vi "CreateImage.vi"() -> ()   [LabVIEW 2020]
panel:
  in  "NumTriangles":i32
  in  "NumImages":i32
  in  "CreateNegImages":bool
  in  "CreatePosImages":bool
  in  "ExportNeg":bool
  in  "NumOvals":i32
  in  "NumRectangles":i32
  in  "stop":bool
  in  "ExportPos":bool
  in  "CreateImage":bool
  out "height":dbl
  out "y":dbl
  out "width":dbl
  out "x":dbl
  out "2D Picture":picture
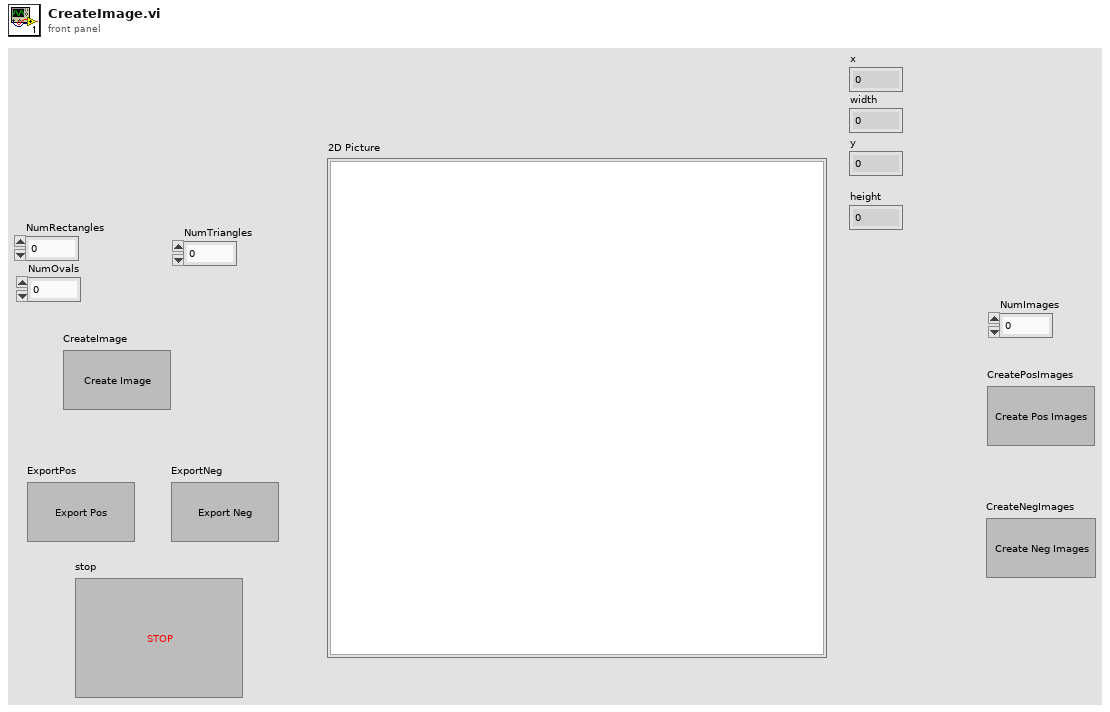
[diagram p1: front panel]
types:
  T1 = cluster{"left":i16, "top":i16, "right":i16, "bottom":i16}
  T2 = enum16{"open", "replace", "create", "open or create", "replace or create", "replace or create with confirmation"}
  T3 = cluster{"Width":u16, "Style":enum32{"Solid", "Dash", "Dot", "DashDot", "DashDotDot"}}
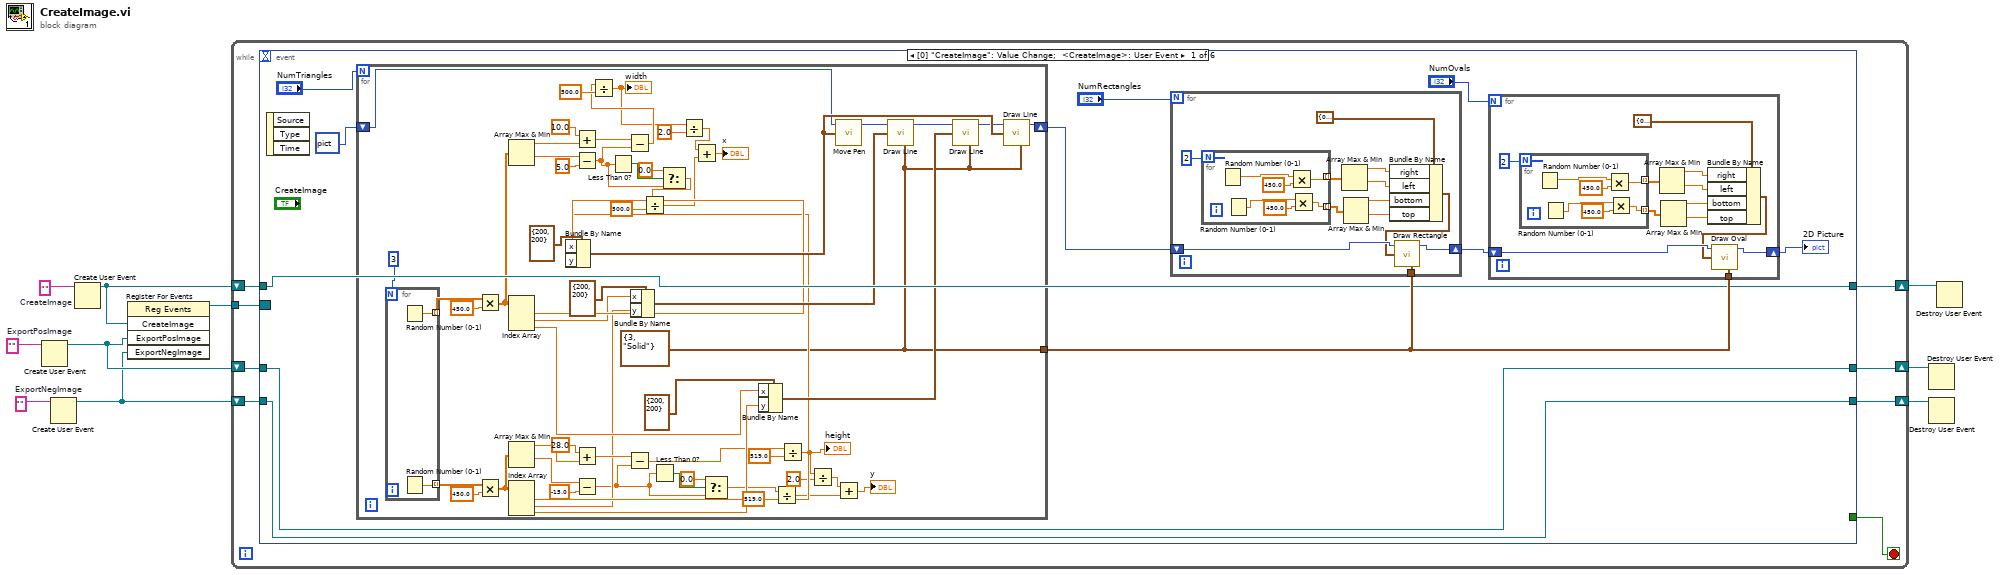
[diagram p0: block diagram]
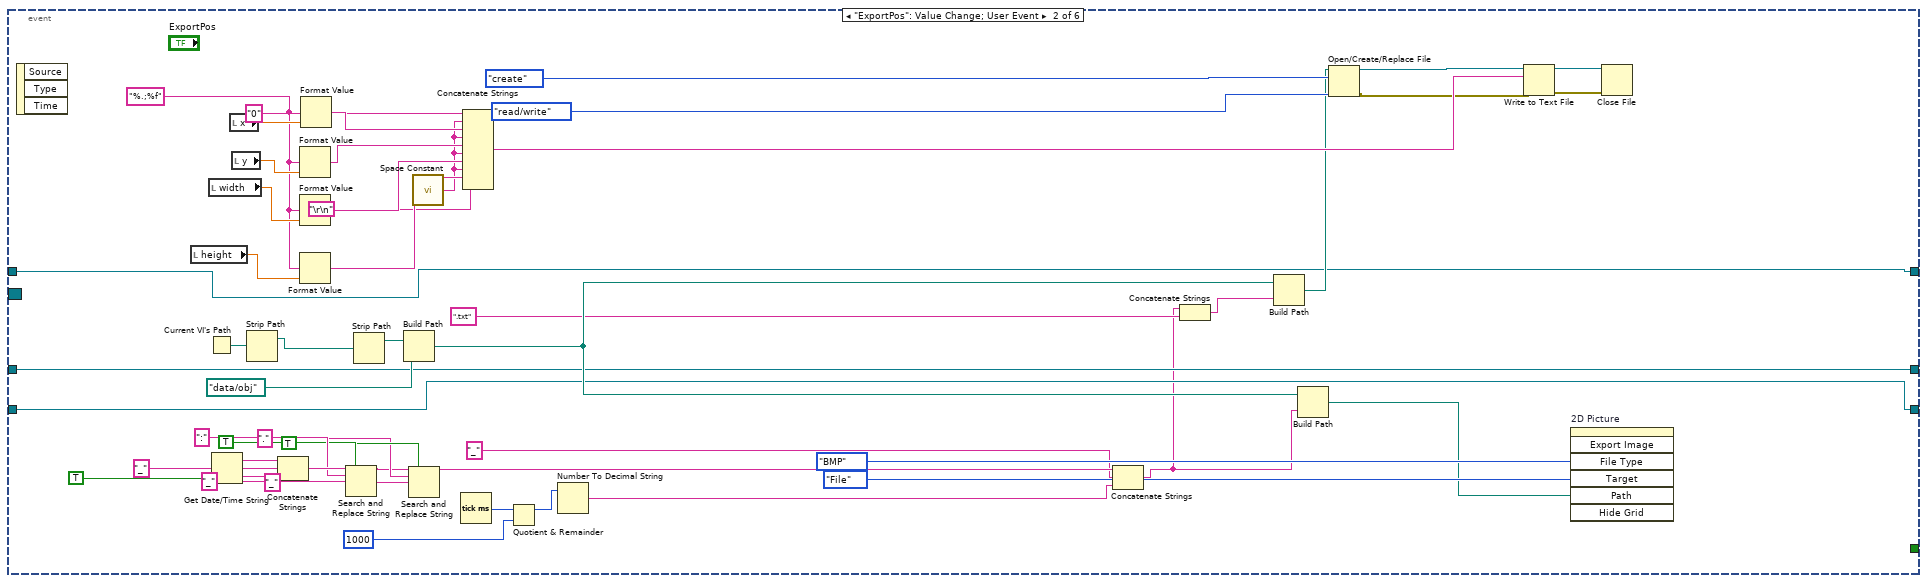
[diagram p2: hidden frame]
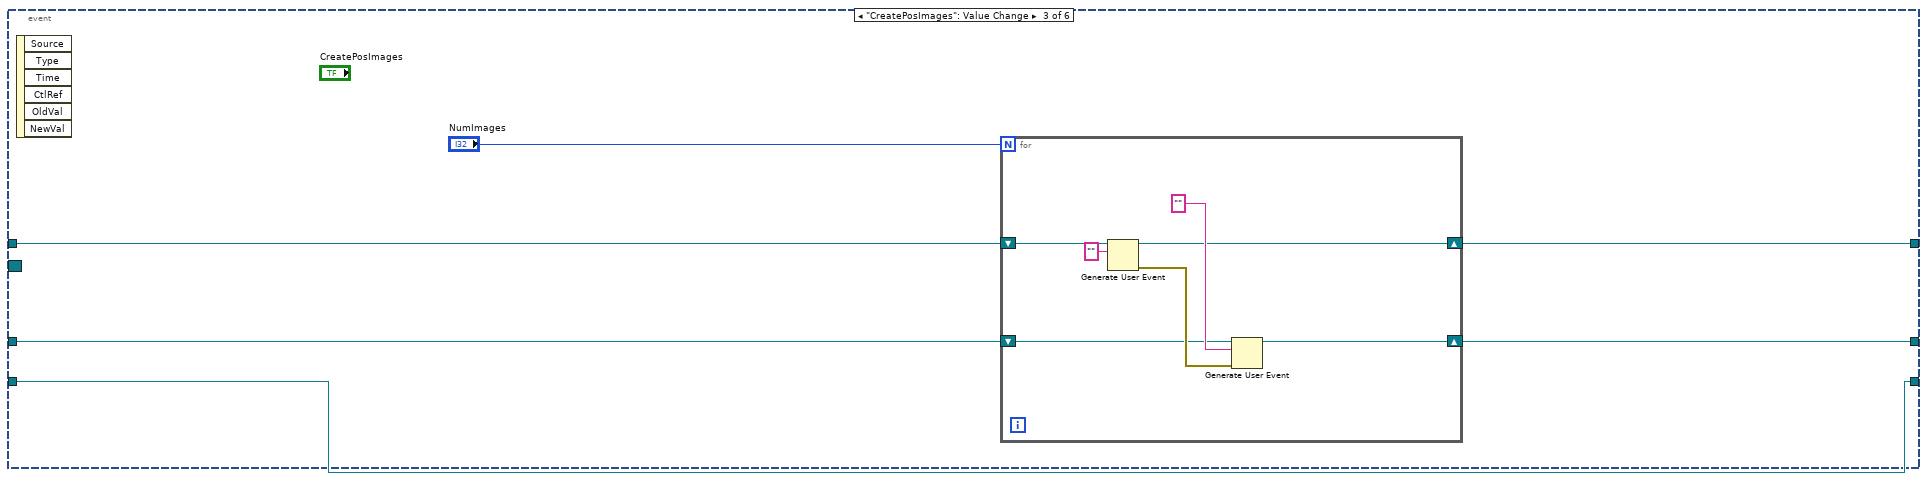
[diagram p3: hidden frame]
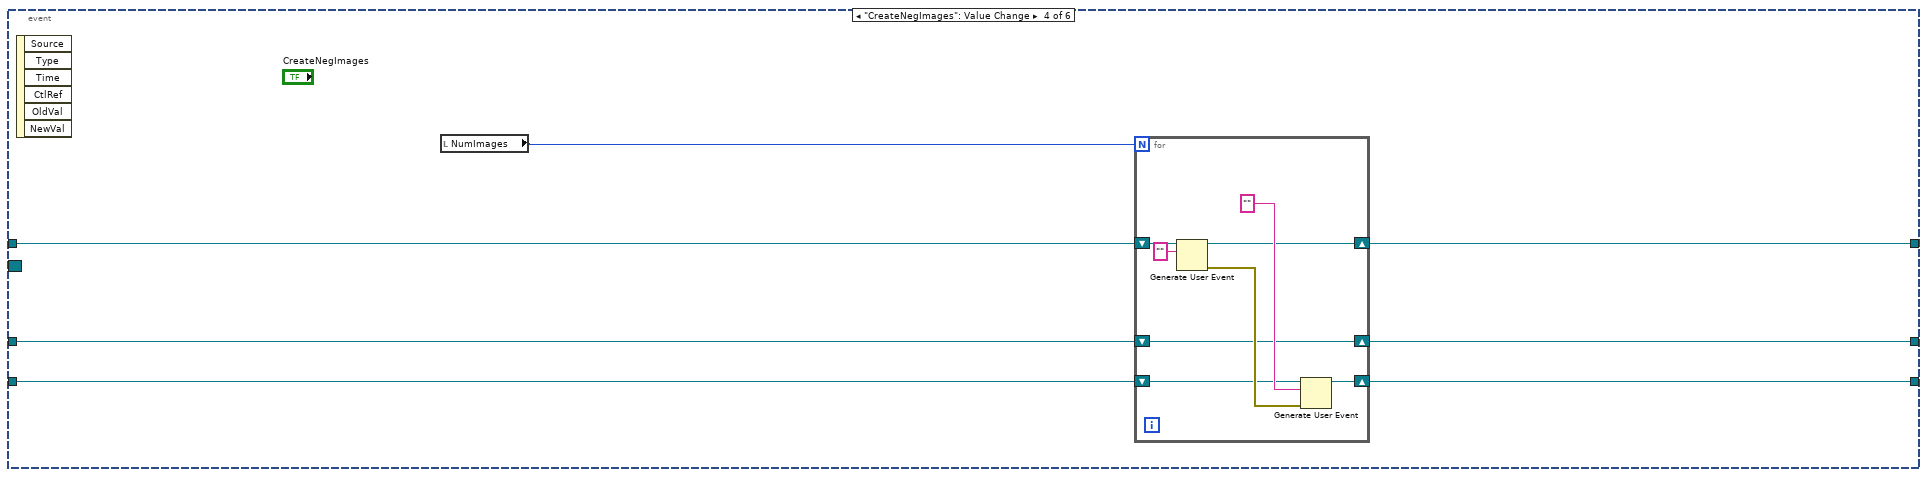
[diagram p4: hidden frame]
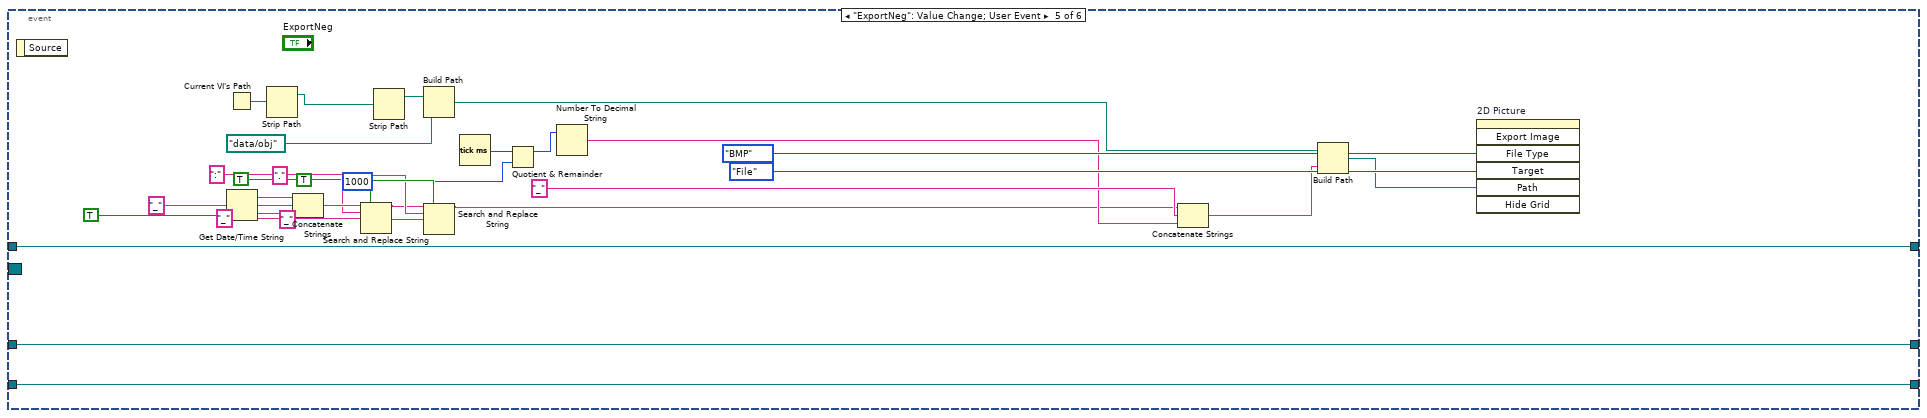
[diagram p5: hidden frame]
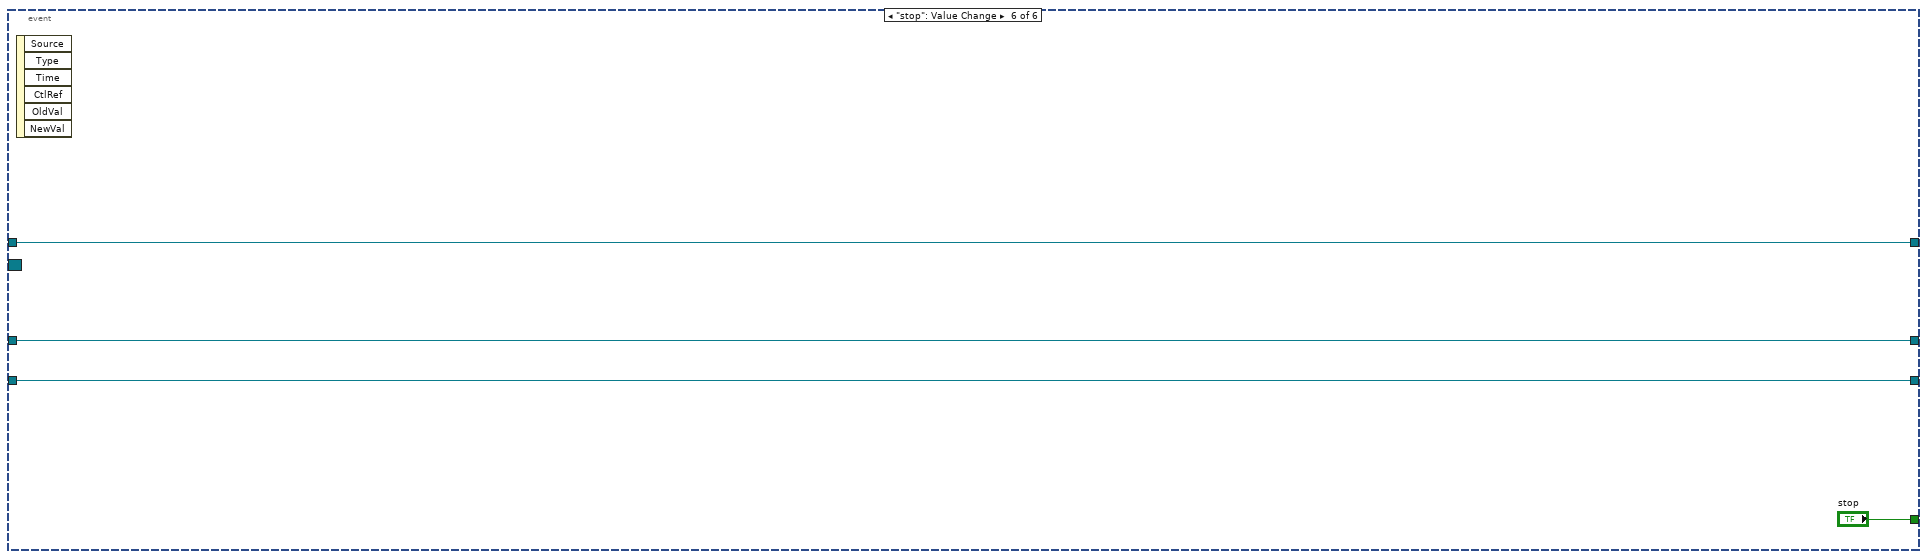
[diagram p6: hidden frame]
diagram:
  w4 = ""  # ExportNegImage
  w6 = ""  # ExportPosImage
  w10 = ""  # CreateImage
  n1 = Create User Event(user event datatype=w6) -> (user event=w5:refnum<user-event>)  [unwired: 1 in, 1 out]
  n2 = Create User Event(user event datatype=w4) -> (user event=w3:refnum<user-event>)  [unwired: 1 in, 1 out]
  n3 = Create User Event(user event datatype=w10) -> (user event=w8:refnum<user-event>)  [unwired: 1 in, 1 out]
  n4 = register-events(w8, w5, w3) -> (reference out=w9:refnum<event-registration>)  [unwired: 2 in, 1 out]
  n5 = while {
    tunnel: w9 -> [w17]
    shift-right: [w15] -> w7
    shift-left: w8 -> [w16]
    shift-right: [w13] -> w2
    shift-left: w5 -> [w14]
    shift-right: [w11] -> w1
    shift-left: w3 -> [w12]
    stop <- w18 stop-if-true
    n6 = event shown="[0] \"CreateImage\": Value Change;  <CreateImage>: User Event" {
      selector: w17 -> [_ _ _ _ _ _]
      dyn-events: _ -> [_ _ _ _ _ _]
      timeout: _ -> [_ _ _ _ _ _]
      tunnel: [_ _ _ _ _ "stop"] -> w18
      tunnel: w16 -> [w23 w134 w184 w198 w216 w239]
      tunnel: [w23 w134 w183 w197 w216 w239] -> w15
      tunnel: w14 -> [w24 w135 w181 w195 w215 w238]
      tunnel: [w24 w135 w182 w196 w215 w238] -> w13
      tunnel: w12 -> [w25 w136 w180 w194 w214 w237]
      tunnel: [w25 w136 w180 w193 w214 w237] -> w11
      event "CreateImage": Value Change; User Event {
        n7 = event-data() -> ()  [unwired: 1 in, 3 out]
        n8 = for {
          N: "NumTriangles" -> [_]
          tunnel: [w59] -> w28
          shift-right: [w34] -> w22
          shift-left: picture data[5B] ("picture") -> [w30]
          w59 = T3 {"Width"=3, "Style"=enum."Solid"} ("pen")
          n9 = for {
            N: 3 -> [_]
            tunnel: [w90] -> w81 mode=indexing
            tunnel: [w89] -> w78 mode=indexing
            n10 = Random Number (0-1)() -> (number: 0 to 1=w90:dbl)
            n11 = Random Number (0-1)() -> (number: 0 to 1=w89:dbl)
          }
          n12 = Multiply(x=w81, y=450.0) -> (x*y=w77:dbl[])
          n13 = Multiply(x=w78, y=450.0) -> (x*y=w67:dbl[])
          n14 = Array Max & Min(array=w77) -> (max value=w74:dbl, min value=w76:dbl)  [unwired: 2 out]
          n15 = Index Array(array=w77) -> (element #1=w65:dbl, element #2=w64:dbl, element #3=w63:dbl)  [unwired: 3 in]
          n16 = Array Max & Min(array=w67) -> (max value=w69:dbl, min value=w68:dbl)  [unwired: 2 out]
          n17 = Index Array(array=w67) -> (element #1=w62:dbl, element #2=w61:dbl, element #3=w60:dbl)  [unwired: 3 in]
          n18 = Bundle By Name(cluster=cluster{"x":i16, "y":i16} {"x"=200, "y"=200} ("new position"), "x"=w65, "y"=w62) -> (w83:cluster{"x":i16, "y":i16})
          n19 = Add(x=10.0, y=w74) -> (x+y=w72:dbl)
          n20 = Subtract(x=w76, y=5.0) -> (x-y=w46:dbl)
          n21 = Add(x=28.0, y=w69) -> (x+y=w71:dbl)
          n22 = Subtract(x=w68, y=-15.0) -> (x-y=w51:dbl)
          n23 = Less Than 0?(x=w46) -> (x < 0?=w48:bool)
          n24 = Subtract(x=w72, y=w46) -> (x-y=w54:dbl)
          n25 = Divide(x=w54, y=500.0) -> (x/y=w39:dbl)
          "width" <- w39
          n26 = Subtract(x=w71, y=w51) -> (x-y=w58:dbl)
          n27 = Bundle By Name(cluster=cluster{"x":i16, "y":i16} {"x"=200, "y"=200} ("new position"), "x"=w64, "y"=w61) -> (w86:cluster{"x":i16, "y":i16})
          n28 = Less Than 0?(x=w51) -> (x < 0?=w52:bool)
          n29 = Select(t=0.0, s=w48, f=w46) -> (s? t:f=w45:dbl)
          n30 = Divide(x=w45, y=500.0) -> (x/y=w36:dbl)
          n31 = Divide(x=w39, y=2.0) -> (x/y=w35:dbl)
          n32 = Add(x=w35, y=w36) -> (x+y=→"x":dbl)
          n33 = Select(t=0.0, s=w52, f=w51) -> (s? t:f=w49:dbl)
          n34 = Bundle By Name(cluster=cluster{"x":i16, "y":i16} {"x"=200, "y"=200} ("new position"), "x"=w63, "y"=w60) -> (w85:cluster{"x":i16, "y":i16})
          n35 = Divide(x=w49, y=519.0) -> (x/y=w44:dbl)
          n36 = Divide(x=w58, y=519.0) -> (x/y=w43:dbl)
          "height" <- w43
          n37 = Divide(x=w43, y=2.0) -> (x/y=w41:dbl)
          n38 = call <vilib>:"Move Pen.vi"("new position"=w83, "picture"=w30) -> ("new picture"=w33:picture)  [unwired: 3 in]
          n39 = Add(x=w41, y=w44) -> (x+y=→"y":dbl)
          n40 = call <vilib>:"Draw Line.vi"("picture"=w33, "end point"=w86, "pen"=w59) -> ("new picture"=w32:picture)  [unwired: 6 in]
          n41 = call <vilib>:"Draw Line.vi"("picture"=w32, "end point"=w85, "pen"=w59) -> ("new picture"=w31:picture)  [unwired: 6 in]
          n42 = call <vilib>:"Draw Line.vi"("picture"=w31, "end point"=w83, "pen"=w59) -> ("new picture"=w34:picture)  [unwired: 6 in]
        }
        n43 = for {
          N: "NumRectangles" -> [_]
          shift-right: [w111] -> w29
          shift-left: w22 -> [w112]
          tunnel: w28 -> [w109]
          n44 = for {
            N: 2 -> [_]
            tunnel: [w124] -> w118 mode=indexing
            tunnel: [w123] -> w117 mode=indexing
            n45 = Random Number (0-1)() -> (number: 0 to 1=w122:dbl)
            n46 = Random Number (0-1)() -> (number: 0 to 1=w121:dbl)
            n47 = Multiply(x=w122, y=450.0) -> (x*y=w124:dbl)
            n48 = Multiply(x=w121, y=450.0) -> (x*y=w123:dbl)
          }
          n49 = Array Max & Min(array=w118) -> (max value=w116:dbl, min value=w115:dbl)  [unwired: 2 out]
          n50 = Array Max & Min(array=w117) -> (max value=w114:dbl, min value=w113:dbl)  [unwired: 2 out]
          n51 = Bundle By Name(cluster=T1 {"left"=0, "top"=0, "right"=0, "bottom"=0} ("rect"), "right"=w116, "left"=w115, "bottom"=w114, "top"=w113) -> (w110:T1)
          n52 = call <vilib>:"Draw Rectangle.vi"("picture"=w112, "rect"=w110, "pen"=w109) -> ("new picture"=w111:picture)  [unwired: 6 in]
        }
        n53 = for {
          N: "NumOvals" -> [_]
          shift-right: [w93] -> w26
          shift-left: w29 -> [w94]
          tunnel: w28 -> [w91]
          n54 = for {
            N: 2 -> [_]
            tunnel: [w106] -> w100 mode=indexing
            tunnel: [w105] -> w99 mode=indexing
            n55 = Random Number (0-1)() -> (number: 0 to 1=w104:dbl)
            n56 = Random Number (0-1)() -> (number: 0 to 1=w103:dbl)
            n57 = Multiply(x=w104, y=450.0) -> (x*y=w106:dbl)
            n58 = Multiply(x=w103, y=450.0) -> (x*y=w105:dbl)
          }
          n59 = Array Max & Min(array=w100) -> (max value=w98:dbl, min value=w97:dbl)  [unwired: 2 out]
          n60 = Array Max & Min(array=w99) -> (max value=w96:dbl, min value=w95:dbl)  [unwired: 2 out]
          n61 = Bundle By Name(cluster=T1 {"left"=0, "top"=0, "right"=0, "bottom"=0} ("rect"), "right"=w98, "left"=w97, "bottom"=w96, "top"=w95) -> (w92:T1)
          n62 = call <vilib>:"Draw Oval.vi"("picture"=w94, "rect"=w92, "pen"=w91) -> ("new picture"=w93:picture)  [unwired: 6 in]
        }
        "2D Picture" <- w26
      }
      event "ExportPos": Value Change; User Event {
        w137 = "%.;%f" ("format string")
        n63 = event-data() -> ()  [unwired: 1 in, 3 out]
        n64 = local read "height"() -> (w140:dbl)
        n65 = Current VI's Path() -> (path=w155:path)
        n66 = local read "width"() -> (w139:dbl)
        n67 = Get Date/Time String(want seconds? (F)=TRUE) -> (date string=w176:string, time string=w175:string)  [unwired: 2 in]
        n68 = local read "x"() -> (w141:dbl)
        n69 = local read "y"() -> (w138:dbl)
        n70 = Strip Path(path=w155) -> (stripped path=w142:path)  [unwired: 1 out]
        n71 = Concatenate Strings(w176, "_" ("string"), w175) -> (w168:string)
        n72 = Format Value(format string=w137, value (0)=w138) -> (output string=w171:string)  [unwired: 1 in]
        n73 = Format Value(format string=w137, value (0)=w139) -> (output string=w170:string)  [unwired: 1 in]
        n74 = Format Value(format string=w137, value (0)=w140) -> (output string=w169:string)  [unwired: 1 in]
        n75 = Format Value(format string=w137, value (0)=w141) -> (output string=w172:string)  [unwired: 1 in]
        n76 = Search and Replace String(replace all?=TRUE ("replace all? (F)"), input string=w168, search string=":", replace string="_" ("replace string (\"\")")) -> (result string=w161:string)  [unwired: 4 in, 3 out]
        n77 = Strip Path(path=w142) -> (stripped path=w150:path)  [unwired: 1 out]
        n78 = Build Path(base path=w150, name or relative path=path "data/obj") -> (appended path=w148:path)
        n79 = Search and Replace String(replace all?=TRUE ("replace all? (F)"), input string=w161, search string=".", replace string="_" ("replace string (\"\")")) -> (result string=w131:string)  [unwired: 4 in, 3 out]
        n80 = call <vilib>:"Space Constant.vi"() -> ("String"=w152:string)
        n81 = Tick Count (ms)() -> (millisecond timer value=w133:u32)
        n82 = Concatenate Strings("0" ("string"), w152, w172, w152, w171, w152, w170, w152, w169, "\r\n") -> (w154:string)
        n83 = Quotient & Remainder(x=w133, y=u32 1000) -> (x-y*floor(x/y)=w128:u32)  [unwired: 1 out]
        n84 = Number To Decimal String(number=w128) -> (decimal integer string=w129:string)  [unwired: 1 in]
        n85 = Concatenate Strings(w131, "_" ("string"), w129) -> (w127:string)
        n86 = Concatenate Strings(w127, ".txt" ("string")) -> (w146:string)
        n87 = Build Path(base path=w148, name or relative path=w146) -> (appended path=w145:path)
        n88 = Build Path(base path=w148, name or relative path=w127) -> (appended path=w173:path)
        n89 = Open/Create/Replace File(file path (use dialog)=w145, operation (0:open)=T2."create", access (0:read/write)=enum16{"read/write", "read-only", "write-only"}."read/write") -> (refnum out=w144:refnum<file>, error out=w143:errorcluster)  [unwired: 3 in, 1 out]
        n90 = Write to Text File(file (use dialog)=w144, text=w154, error in=w143) -> (refnum out=w159:refnum<file>, error out=w158:errorcluster)  [unwired: 1 in, 1 out]
        n91 = invoke on="2D Picture" class="Pict" method="Export Image"("File Type"=enum32{"BMP", "EPS", "EMF", "PICT"}."BMP", "Target"=enum32{"File", "Clipboard"}."File", "Path"=w173) -> ()  [unwired: 4 in, 7 out]
        n92 = Close File(refnum=w159, error in=w158) -> ()  [unwired: 2 out]
      }
      event "CreatePosImages": Value Change {
        n93 = event-data() -> ()  [unwired: 1 in, 6 out]
        n94 = for {
          N: "NumImages" -> [_]
          shift-right: [w186] -> w183
          shift-left: w184 -> [w191]
          shift-right: [w185] -> w182
          shift-left: w181 -> [w187]
          n95 = Generate User Event(user event=w191, event data cluster="" ("event data")) -> (user event out=w186:refnum<user-event>, error out=w188:errorcluster)  [unwired: 2 in]
          n96 = Generate User Event(user event=w187, event data cluster="" ("event data"), error in=w188) -> (user event out=w185:refnum<user-event>)  [unwired: 1 in, 1 out]
        }
      }
      event "CreateNegImages": Value Change {
        n97 = event-data() -> ()  [unwired: 1 in, 6 out]
        n98 = local read "NumImages"() -> (w192:i32)
        n99 = for {
          N: w192 -> [_]
          shift-right: [w202] -> w197
          shift-left: w198 -> [w206]
          shift-right: [w200] -> w196
          shift-left: w195 -> [w200]
          shift-right: [w199] -> w193
          shift-left: w194 -> [w201]
          n100 = Generate User Event(user event=w206, event data cluster="" ("event data")) -> (user event out=w202:refnum<user-event>, error out=w203:errorcluster)  [unwired: 2 in]
          n101 = Generate User Event(user event=w201, event data cluster="" ("event data"), error in=w203) -> (user event out=w199:refnum<user-event>)  [unwired: 1 in, 1 out]
        }
      }
      event "ExportNeg": Value Change; User Event {
        n102 = event-data() -> ()  [unwired: 1 in, 1 out]
        n103 = Current VI's Path() -> (path=w222:path)
        n104 = Get Date/Time String(want seconds? (F)=TRUE) -> (date string=w234:string, time string=w233:string)  [unwired: 2 in]
        n105 = Strip Path(path=w222) -> (stripped path=w218:path)  [unwired: 1 out]
        n106 = Concatenate Strings(w234, "_" ("string"), w233) -> (w231:string)
        n107 = Search and Replace String(replace all?=TRUE ("replace all? (F)"), input string=w231, search string=":", replace string="_" ("replace string (\"\")")) -> (result string=w224:string)  [unwired: 4 in, 3 out]
        n108 = Strip Path(path=w218) -> (stripped path=w221:path)  [unwired: 1 out]
        n109 = Build Path(base path=w221, name or relative path=path "data/obj") -> (appended path=w219:path)
        n110 = Search and Replace String(replace all?=TRUE ("replace all? (F)"), input string=w224, search string=".", replace string="_" ("replace string (\"\")")) -> (result string=w208:string)  [unwired: 4 in, 3 out]
        n111 = Tick Count (ms)() -> (millisecond timer value=w213:u32)
        n112 = Quotient & Remainder(x=w213, y=u32 1000) -> (x-y*floor(x/y)=w209:u32)  [unwired: 1 out]
        n113 = Number To Decimal String(number=w209) -> (decimal integer string=w210:string)  [unwired: 1 in]
        n114 = Concatenate Strings(w208, "_" ("string"), w210) -> (w207:string)
        n115 = Build Path(base path=w219, name or relative path=w207) -> (appended path=w217:path)
        n116 = invoke on="2D Picture" class="Pict" method="Export Image"("File Type"=enum32{"BMP", "EPS", "EMF", "PICT"}."BMP", "Target"=enum32{"File", "Clipboard"}."File", "Path"=w217) -> ()  [unwired: 4 in, 7 out]
      }
      event "stop": Value Change {
        n117 = event-data() -> ()  [unwired: 1 in, 6 out]
      }
    }
  }
  n118 = Destroy User Event(user event=w2) -> ()  [unwired: 1 in, 1 out]
  n119 = Destroy User Event(user event=w1) -> ()  [unwired: 1 in, 1 out]
  n120 = Destroy User Event(user event=w7) -> ()  [unwired: 1 in, 1 out]
